vi "gxml_WriteXMLtoFile.vi"(8 "error in":errorcluster, 10 "XML Input":string, 11 "XML File Path":path) -> (0 "error out":errorcluster, 3 "XML File Path Out":path)   [LabVIEW 2011, in "Third Party VIs.lvlib" / "GXML.lvlib"]
doc: "This VI prepends the input string with an XML file header and writes everything to a text file with an XML extension."
uses:
  GXML.lvlib
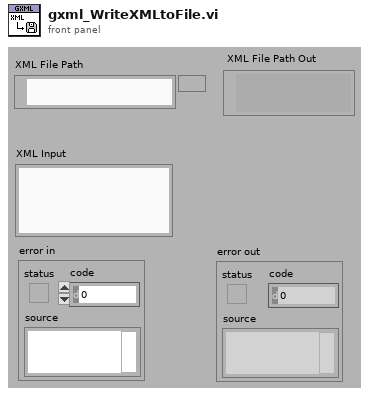
[diagram p1: front panel]
types:
  T1 = enum16{"open", "replace", "create", "open or create", "replace or create", "replace or create with confirmation"}
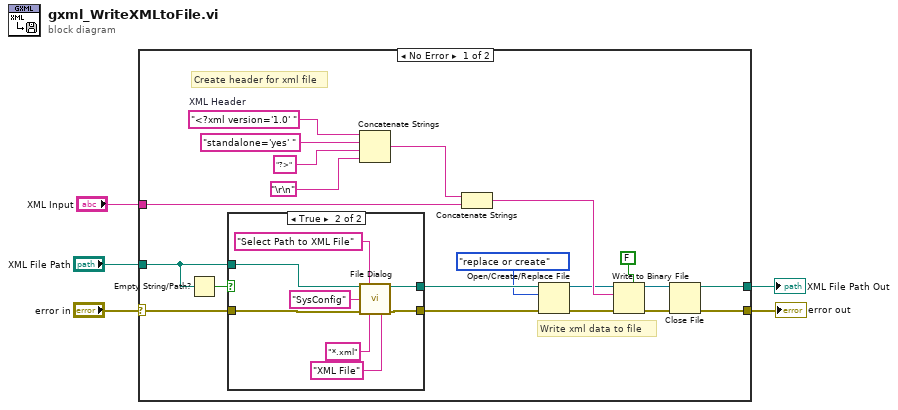
[diagram p0: block diagram]
diagram:
  n1 = case shown="No Error" "error in" {
    selector: "error in" -> [w14 w37]
    tunnel: [w19 w37] -> w4
    tunnel: "XML Input" -> [w21 _]
    tunnel: "XML File Path" -> [w8 w36]
    tunnel: [w6 w36] -> w1
    frame No Error {
      w25 = "<?xml version='1.0' "  # XML Header
      # "Create header for xml file"
      # "Write xml data to file"
      n2 = Empty String/Path?(string/path=w8) -> (empty?=w7:bool)
      n3 = case shown="True" w7 {
        tunnel: w14 -> [w27 w35]
        tunnel: [w26 w30] -> w11
        tunnel: [w27 w29] -> w10
        tunnel: w8 -> [w26 w28]
        frame False {
        }
        frame True {
          n4 = call "File Dialog"("start path"=w28, "prompt"="Select Path to XML File" ("Prompt"), "default name"="SysConfig", "error in"=w35, "pattern (all files)"="*.xml" ("pattern"), "pattern label"="XML File") -> ("selected path"=w30:path, "error out"=w29:errorcluster)  [unwired: 6 in, 2 out]
        }
      }
      n5 = Concatenate Strings(w25, "standalone='yes' " ("Substring"), "?>" ("Substring"), "\r\n") -> (w23:string)
      n6 = Concatenate Strings(w23, w21) -> (w18:string)
      n7 = Open/Create/Replace File(file path (use dialog)=w11, error in=w10, operation (0:open)=T1."replace or create") -> (refnum out=w13:refnum<file>, error out=w12:errorcluster)  [unwired: 3 in, 1 out]
      n8 = Write to Binary File(file (use dialog)=w13, data=w18, error in=w12, 5:FALSE ("prepend array or string size? (T)")) -> (refnum out=w17:refnum<file>, error out=w20:errorcluster)  [unwired: 3 out]
      n9 = Close File(refnum=w17, error in=w20) -> (path=w6:path, error out=w19:errorcluster)
    }
    frame Error {
    }
  }
  "error out" <- w4
  "XML File Path Out" <- w1
